vi "DAQmx.Enumerate And Sort Devices.vi"(8 "error in (no error)":errorcluster, 11 "DAQmx in":refnum<class "DAQmx.lvclass">) -> (0 "error out":errorcluster, 2 "Devices (sorted)":T1[](array[typedef]), 3 "DAQmx out":refnum<class "DAQmx.lvclass">)   [LabVIEW 2019, in "DAQmx.lvclass"]
uses:
  DAQmx.lvclass
  typedefs/DeviceInfo--Cluster.ctl
  DAQmx.lvclass/DAQmx.ctl
  <vilib>/numeric/Random Number (Range) I64.vi
  <vilib>/numeric/sub_Random U32.vi
  <userlib>/_OpenG.lib/array/array.llb/Sort 1D Array (U32)__ogtk.vi
  <userlib>/_OpenG.lib/array/array.llb/Reorder 1D Array2 (Variant)__ogtk.vi
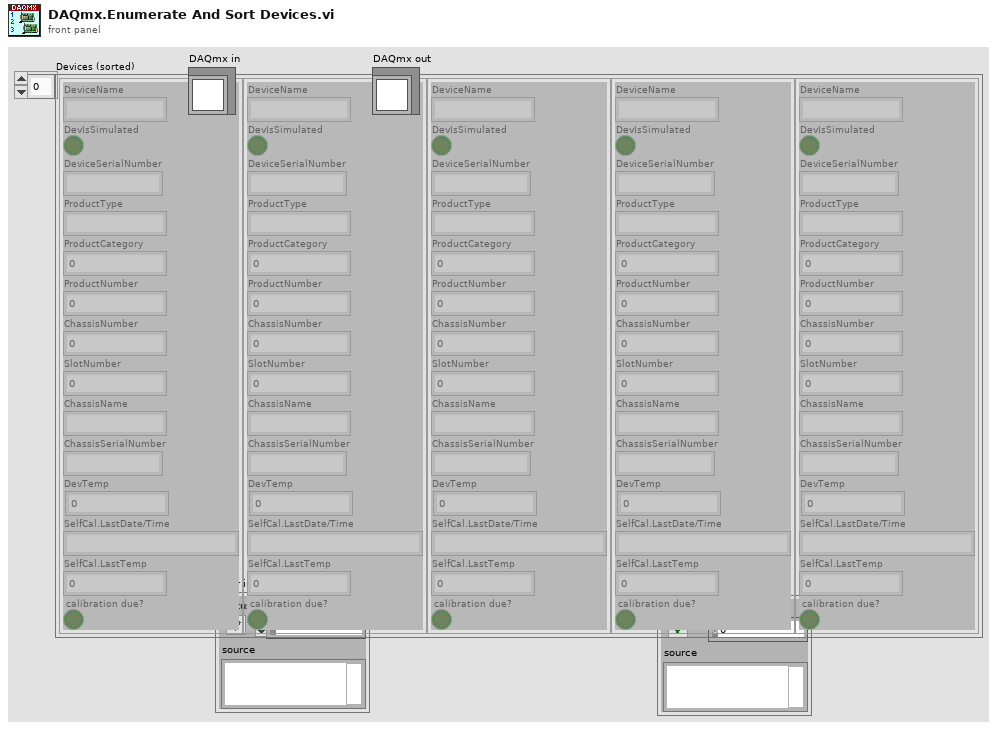
[diagram p1: front panel]
types:
  T1 = typedef "DAQmx.lvclass/DeviceInfo--Cluster.ctl" = cluster{"DeviceName":string, "DevIsSimulated":bool, "DeviceSerialNumber":string, "ProductType":string, "ProductCategory":i32, "ProductNumber":u32, "ChassisNumber":u32, "SlotNumber":u32, "ChassisName":string, "ChassisSerialNumber":string, "DevTemp":dbl, "SelfCal.LastDate/Time":string, "SelfCal.LastTemp":dbl, "calibration due?":bool}
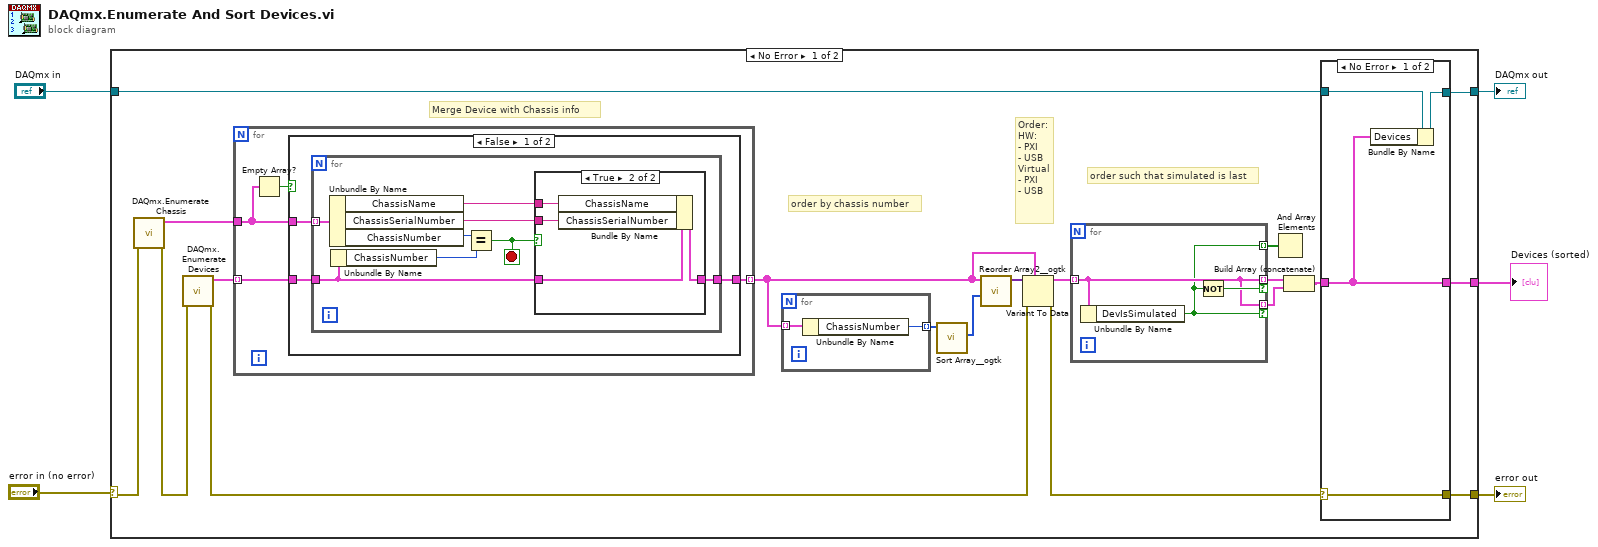
[diagram p0: block diagram]
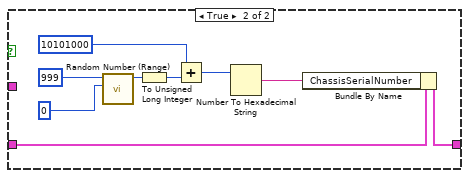
[diagram p3: hidden frame]
diagram:
  n1 = case shown="No Error" "error in (no error)" {
    selector: "error in (no error)" -> [w11 w66]
    tunnel: [w8 w66] -> w4
    tunnel: "DAQmx in" -> [w14 w65]
    tunnel: [w7 w65] -> w2
    tunnel: [w6 _] -> w1
    frame No Error {
      # "Order:\nHW:\n- PXI\n- USB\nVirtual\n- PXI\n- USB"
      # "order by chassis number"
      # "order such that simulated is last"
      # "Merge Device with Chassis info"
      n2 = call "DAQmx.Enumerate Chassis.vi"("error in (no error)"=w11) -> ("error out"=w10:errorcluster, "Chassis and Controllers"=w21:T1[])  [unwired: 9 in]
      n3 = call "DAQmx.Enumerate Devices.vi"("error in (no error)"=w10) -> ("error out"=w9:errorcluster, "Devices"=w22:T1[])  [unwired: 9 in]
      n4 = for {
        tunnel: w21 -> [w26]
        tunnel: w22 -> [w27] mode=indexing
        tunnel: [w28] -> w17 mode=indexing
        n5 = Empty Array?(array=w26) -> (empty?=w25:bool)
        n6 = case shown="False" w25 {
          tunnel: [w31 w53] -> w28
          tunnel: w27 -> [w30 w52]
          tunnel: w26 -> [w29 _]
          frame False {
            n7 = for {
              tunnel: w30 -> [w32]
              tunnel: w29 -> [w39] mode=indexing
              tunnel: [w34] -> w31
              stop <- w33 stop-if-true
              n8 = Unbundle By Name(w39) -> ("ChassisName"=w36:string, "ChassisSerialNumber"=w35:string, "ChassisNumber"=w38:u32)
              n9 = Unbundle By Name(w32) -> ("ChassisNumber"=w37:u32)
              n10 = Equal?(x=w38, y=w37) -> (x = y?=w33:bool)
              n11 = case shown="True" w33 {
                tunnel: w32 -> [w40 w44]
                tunnel: w36 -> [_ w43]
                tunnel: w35 -> [_ w41]
                tunnel: [w40 w42] -> w34
                frame False {
                }
                frame True {
                  n12 = Bundle By Name(cluster=w44, "ChassisName"=w43, "ChassisSerialNumber"=w41) -> (w42:T1)
                }
              }
            }
          }
          frame True {
            n13 = call-poly <vilib>:"Random Number (Range).vi"("lower bound (-100)"=i64 0, "upper bound (100)"=i64 999) -> ("number"=w48:i64)  [unwired: 9 in]
            n14 = To Unsigned Long Integer(number=w48) -> (unsigned 32bit integer=w47:u32)
            n15 = Add(x=u32 10101000 ("ChassisSerialNumber"), y=w47) -> (x+y=w46:u32)
            n16 = Number To Hexadecimal String(2:w46) -> (0:w45:string)  [unwired: 1 in]
            n17 = Bundle By Name(cluster=w52, "ChassisSerialNumber"=w45) -> (w53:T1)
          }
        }
      }
      n18 = for {
        tunnel: w17 -> [w58] mode=indexing
        tunnel: [w57] -> w20 mode=indexing
        n19 = Unbundle By Name(w58) -> ("ChassisNumber"=w57:u32)
      }
      n20 = call-poly <userlib>:"Sort Array__ogtk.vi"("Array in"=w20) -> ("Sorted Pointers"=w19:i32[])  [unwired: 9 in, 1 out]
      n21 = call-poly <userlib>:"Reorder Array2__ogtk.vi"("indices"=w19, "array"=w17) -> ("reordered array"=w18:variant[])  [unwired: 9 in]
      n22 = Variant To Data(error in=w9, type=w17, Variant=w18) -> (data=w16:T1[], error out=w15:errorcluster)
      n23 = for {
        tunnel: [w55] -> w24 mode=indexing if=w56
        tunnel: w16 -> [w55] mode=indexing
        tunnel: [w55] -> w23 mode=indexing if=w54
        tunnel: [w54] -> w13 mode=indexing
        n24 = Unbundle By Name(w55) -> ("DevIsSimulated"=w54:bool)
        n25 = Not(x=w54) -> (.not. x?=w56:bool)
      }
      n26 = And Array Elements(Boolean array=w13) -> ()  [unwired: 1 out]
      n27 = Build Array (concatenate)(w24, w23) -> (w12:T1[])
      n28 = case shown="No Error" w15 {
        selector: w15 -> [w60 w64]
        tunnel: [w60 w64] -> w8
        tunnel: w14 -> [w62 w63]
        tunnel: w12 -> [w59 _]
        tunnel: [w61 w63] -> w7
        tunnel: [w59 _] -> w6
        frame No Error {
          n29 = Bundle By Name(cluster=w62, "Devices"=w59) -> (w61:refnum<class "DAQmx.lvclass">)
        }
        frame Error {
        }
      }
    }
    frame Error {
    }
  }
  "error out" <- w4
  "DAQmx out" <- w2
  "Devices (sorted)" <- w1
